vi "limit_plot_size.vi"() -> ()   [LabVIEW 2019]
panel:
  in  "Number of Points to Generate":i32=600000
  in  "Boolean":bool=TRUE
  in  "Reset Zoom?":bool
  out "XYPlot":cluster{dbl[], dbl[]}[](graph)
  out "Decimation Factor":u32
  in  "Number of Points Per Pixel":u32=1
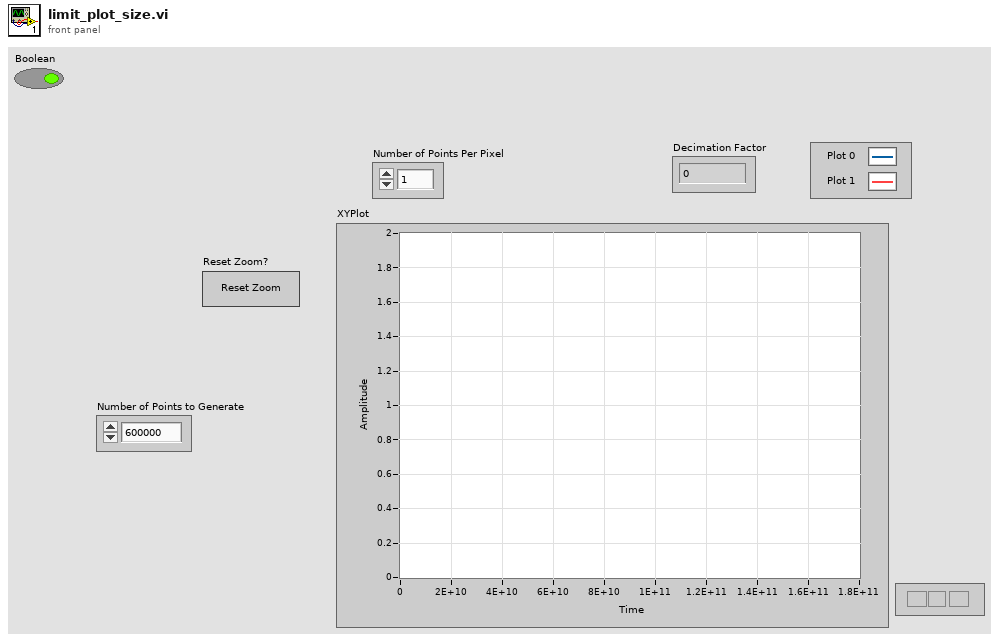
[diagram p1: front panel]
types:
  T1 = typedef "LVRangeTypeDef.ctl" = cluster{"Minimum":dbl, "Maximum":dbl, "Increment":dbl, "Minor Increment":dbl, "Start":dbl}
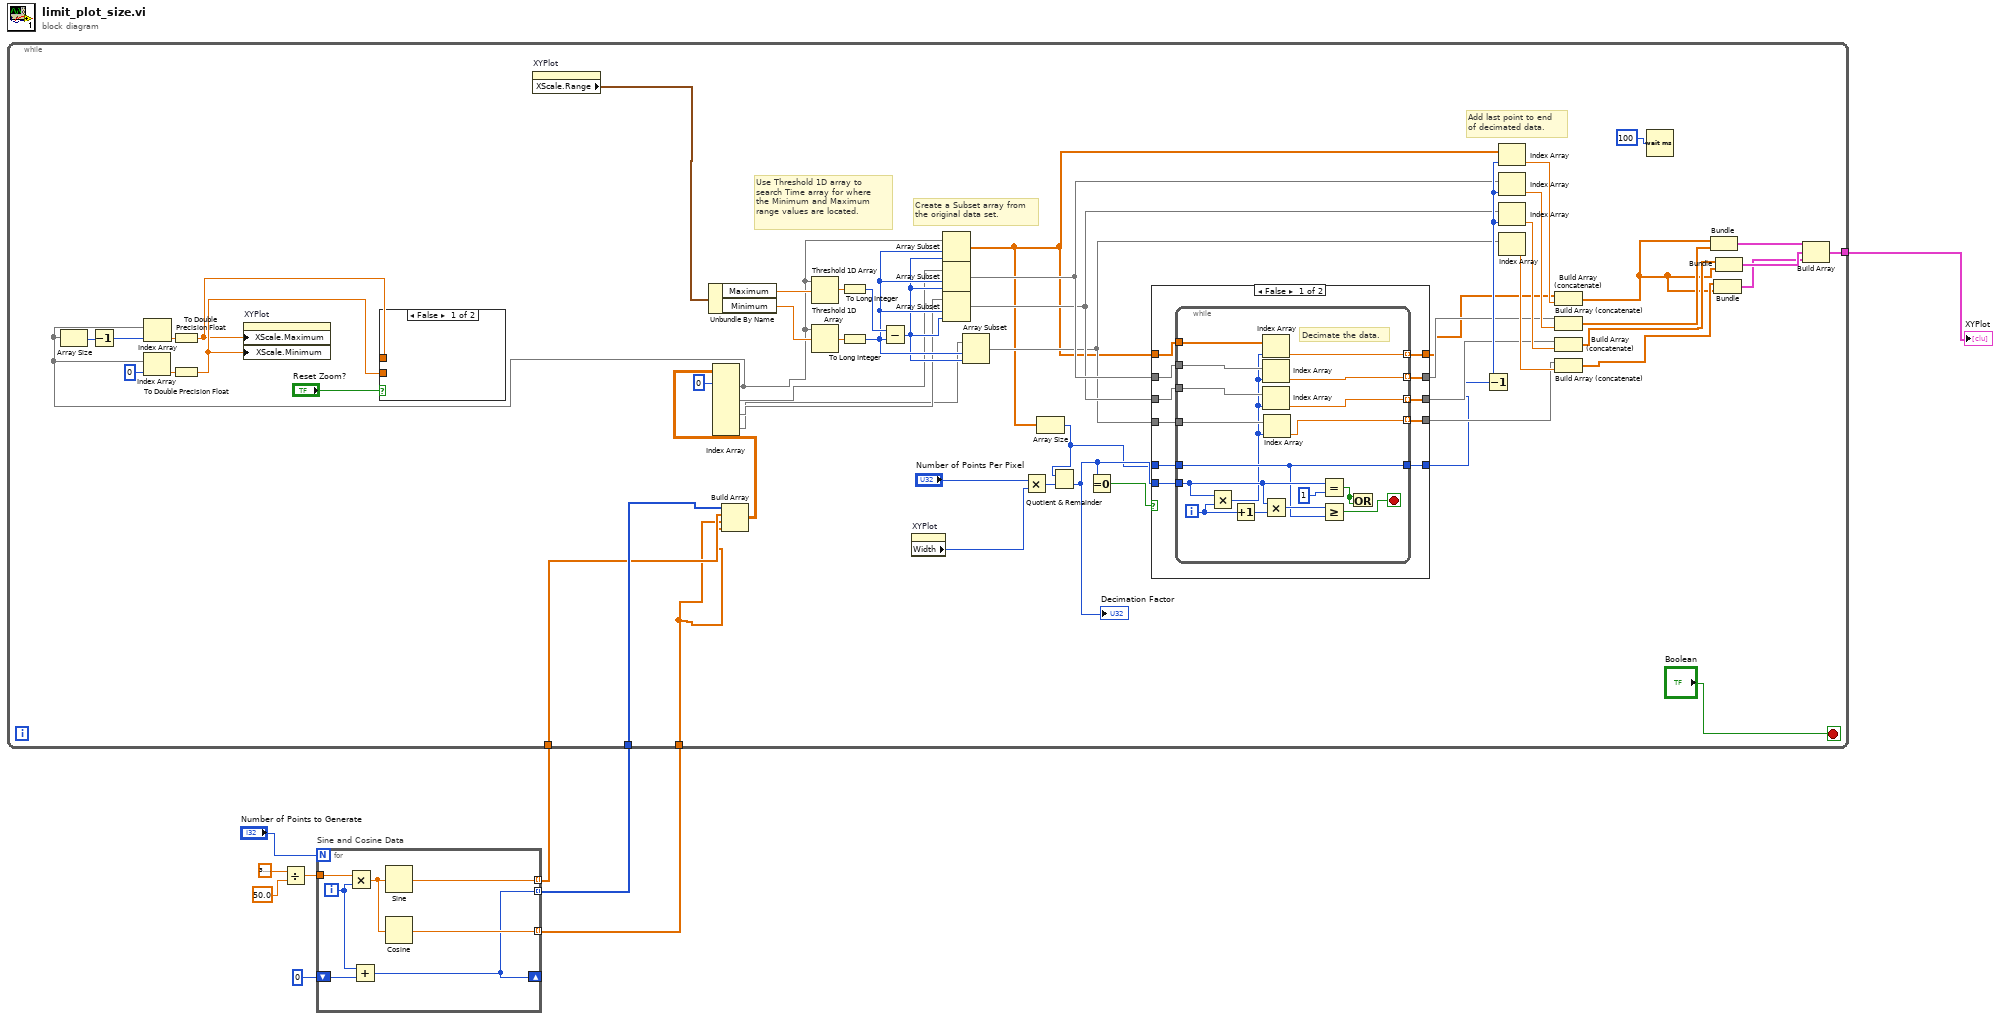
[diagram p0: block diagram]
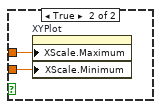
[diagram p2: hidden frame]
diagram:
  n1 = Divide(x=3.141592653589793, y=50.0) -> (x/y=w6:dbl)
  n2 = for "Sine and Cosine Data" {
    N: "Number of Points to Generate" -> [_]
    tunnel: w6 -> [w16]
    tunnel: [w14] -> w2 mode=indexing
    tunnel: [w13] -> w1 mode=indexing
    shift-right: [w10] -> _
    shift-left: i64 0 -> [w12]
    tunnel: [w10] -> w3 mode=indexing
    i -> [w11]
    n3 = Multiply(x=w16, y=w11) -> (x*y=w15:dbl)
    n4 = Add(x=w11, y=w12) -> (x+y=w10:i64)
    n5 = Sine(x=w15) -> (sin(x)=w14:dbl)
    n6 = Cosine(x=w15) -> (cos(x)=w13:dbl)
  }
  n7 = while {
    tunnel: [w22] -> w9
    tunnel: w3 -> [w19]
    tunnel: w2 -> [w18]
    tunnel: w1 -> [w17]
    stop <- "Boolean" stop-if-true
    # "Add last point to end\nof decimated data."
    # "Create a Subset array from\nthe original data set."
    # "Use Threshold 1D array to\nsearch Time array for where\nthe Minimum and Maximum\nrange values are located."
    n8 = property on="XYPlot" class="XYGraph (strict)"() -> ("XScale.Range"=w71:T1)  [unwired: 2 in, 2 out]
    n9 = Unbundle By Name(w71) -> ("Maximum"=w60:dbl, "Minimum"=w64:dbl)
    n10 = Build Array(w19, w18, w17, w17) -> (w33:dbl[][])
    n11 = Index Array(array=w33, index (row) #1=0 ("index")) -> (element #1=w30:dbl[], element #2=w57:dbl[], element #3=w56:dbl[], element #4=w55:dbl[])  [unwired: 7 in]
    n12 = Array Size(array=w30) -> (size(s)=w40:i32)
    n13 = Decrement(x=w40) -> (x-1=w39:i32)
    n14 = Index Array(array=w30, index=0) -> (element=w36:dbl)
    n15 = Index Array(array=w30, index=w39) -> (element=w38:dbl)
    n16 = To Double Precision Float(number=w38) -> (double precision float=w34:dbl)
    n17 = To Double Precision Float(number=w36) -> (double precision float=w35:dbl)
    n18 = property on="XYPlot" class="XYGraph (strict)"("XScale.Maximum"=w34, "XScale.Minimum"=w35) -> ()  [unwired: 2 in, 2 out]
    n19 = case shown="False" "Reset Zoom?" {
      tunnel: w34 -> [_ w73]
      tunnel: w35 -> [_ w72]
      frame False {
      }
      frame True {
        n20 = property on="XYPlot" class="XYGraph (strict)"("XScale.Maximum"=w73, "XScale.Minimum"=w72) -> ()  [unwired: 2 in, 2 out]
      }
    }
    n21 = Threshold 1D Array(2:w60, 3:w30) -> (0:w63:dbl)  [unwired: 1 in]
    n22 = Threshold 1D Array(2:w64, 3:w30) -> (0:w62:dbl)  [unwired: 1 in]
    n23 = To Long Integer(number=w63) -> (32bit integer=w61:i32)
    n24 = To Long Integer(number=w62) -> (32bit integer=w59:i32)
    n25 = Subtract(x=w61, y=w59) -> (x-y=w58:i32)
    n26 = property on="XYPlot" class="XYGraph (strict)"() -> ("Width"=w68:u32)  [unwired: 2 in, 2 out]
    n27 = Array Subset(array=w30, index=w59, length=w58) -> (w32:dbl[])
    n28 = Array Subset(array=w57, index=w59, length=w58) -> (w44:dbl[])
    n29 = Array Subset(array=w56, index=w59, length=w58) -> (w43:dbl[])
    n30 = Array Subset(array=w55, index=w59, length=w58) -> (w42:dbl[])
    n31 = Multiply(x="Number of Points Per Pixel", y=w68) -> (x*y=w70:u32)
    n32 = Array Size(array=w32) -> (size(s)=w31:i32)
    n33 = Quotient & Remainder(x=w31, y=w70) -> (floor(x/y)=w66:u32)  [unwired: 1 out]
    "Decimation Factor" <- w66
    n34 = Equal To 0?(x=w66) -> (x = 0?=w67:bool)
    n35 = case shown="False" w67 {
      tunnel: [w84 w103] -> w45
      tunnel: w32 -> [w83 w106]
      tunnel: w44 -> [w82 w105]
      tunnel: w43 -> [w81 w104]
      tunnel: [w80 w105] -> w47
      tunnel: [w79 w104] -> w48
      tunnel: w31 -> [w74 w103]
      tunnel: [w78 w106] -> w46
      tunnel: w66 -> [w77 _]
      tunnel: w42 -> [w76 w102]
      tunnel: [w75 w102] -> w49
      frame False {
        n36 = while {
          tunnel: w83 -> [w98]
          tunnel: w82 -> [w93]
          tunnel: w81 -> [w97]
          tunnel: w74 -> [w90]
          tunnel: [w96] -> w78 mode=indexing
          tunnel: [w95] -> w80 mode=indexing
          tunnel: [w94] -> w79 mode=indexing
          tunnel: w77 -> [w92]
          tunnel: [w90] -> w84
          tunnel: w76 -> [w87]
          tunnel: [w86] -> w75 mode=indexing
          i -> [w101]
          stop <- w88 stop-if-true
          # "Decimate the data."
          n37 = Multiply(x=w92, y=w101) -> (x*y=w85:u32)
          n38 = Increment(x=w101) -> (x+1=w100:i32)
          n39 = Index Array(array=w98, index=w85) -> (element=w96:dbl)
          n40 = Index Array(array=w93, index=w85) -> (element=w95:dbl)
          n41 = Index Array(array=w97, index=w85) -> (element=w94:dbl)
          n42 = Multiply(x=w92, y=w100) -> (x*y=w99:u32)
          n43 = Index Array(array=w87, index=w85) -> (element=w86:dbl)
          n44 = Equal?(x=w92, y=u32 1) -> (x = y?=w89:bool)
          n45 = Greater Or Equal?(x=w99, y=w90) -> (x >= y?=w88:bool)
          n46 = Or(x=w89, y=w89) -> ()  [unwired: 1 out]
        }
      }
      frame True {
      }
    }
    n47 = Decrement(x=w45) -> (x-1=w54:i32)
    n48 = Index Array(array=w32, index=w54) -> (element=w51:dbl)
    n49 = Index Array(array=w44, index=w54) -> (element=w53:dbl)
    n50 = Index Array(array=w43, index=w54) -> (element=w52:dbl)
    n51 = Index Array(array=w42) -> (element=w50:dbl)  [unwired: 1 in]
    n52 = Build Array (concatenate)(w46, w51) -> (w26:dbl[])
    n53 = Build Array (concatenate)(w47, w53) -> (w29:dbl[])
    n54 = Build Array (concatenate)(w48, w52) -> (w28:dbl[])
    n55 = Build Array (concatenate)(w49, w50) -> (w27:dbl[])
    n56 = Wait (ms)(milliseconds to wait=100) -> ()  [unwired: 1 out]
    n57 = Bundle(w26, w29) -> (w25:cluster{dbl[], dbl[]})  [unwired: 1 in]
    n58 = Bundle(w27, w26) -> (w23:cluster{dbl[], dbl[]})  [unwired: 1 in]
    n59 = Bundle(w28, w26) -> (w24:cluster{dbl[], dbl[]})  [unwired: 1 in]
    n60 = Build Array(w25, w24, w23) -> (w22:cluster{dbl[], dbl[]}[])
  }
  "XYPlot" <- w9
